vi "Library - Description.vi"(7 "Msg Chain":string, 8 "error in (no error)":errorcluster {"code" format="Error %.0f"}, 10 "Libraries":refnum<class "Library Documentation.lvclass">[](array[class]), 11 "VIDoc Printer - Confluence In":refnum<class "VIDoc Printer - Confluence.lvclass">) -> (0 "error out":errorcluster {"code" format="Error %.0f"}, 3 "VIDoc Printer - Confluence Out":refnum<class "VIDoc Printer - Confluence.lvclass">)   [LabVIEW 2023, in "VIDoc Printer - Confluence.lvlib" / "VIDoc Printer - Confluence.lvclass"]
uses:
  VIDoc Printer - Confluence.lvclass
  C:/projects/DMC/Tooling/Git-Action-Service/Source/Documentation Generation/Printers/Printer/VIDoc Printer.lvclass
  Parsing/Library Documentation/Library Documentation.lvclass
  Parsing/Library Documentation/Library Documentation.lvclass/Library Documentation.ctl
  Parsing/Library Documentation/Get Library Info.vi
  Parsing/Library Documentation/Get Name.vi
  VIDoc Printer - Confluence.lvclass/VIDoc Printer - Confluence.ctl
  Printer/VIDoc Printer.lvclass
  UI Interaction/UI Interaction.lvclass
  C:/projects/DMC/Tooling/Git-Action-Service/Source/Documentation Generation/Printers/Confluence Printer/VIDoc Printer - Confluence.lvclass
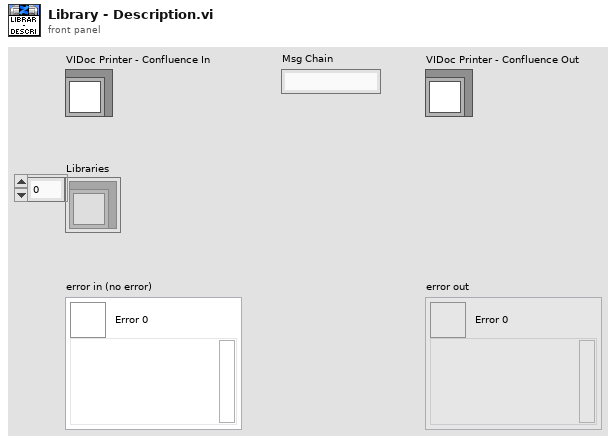
[diagram p1: front panel]
types:
  T1 = typedef "VIDoc Parsing.lvlib/Base Library Info Cluster.ctl" = cluster{"Name":string, "Icon":T2, "Version":cluster{"Major":u16, "Minor":u16, "Fix":u16, "Build":u16}, "Description":string, "Path":path, "Friends":string[], "Library Scope":enum32{"invalid scope", "public", "private", "protected", "community"}, "Qualified Name":string}
  T2 = typedef "imagedata.ctl" = cluster{"image type":i32, "image depth":i32, "image":u8[], "mask":u8[], "colors":u32[], "Rectangle":cluster{"left":i16, "top":i16, "right":i16, "bottom":i16}}
  T3 = enum32{"invalid scope", "public", "private", "protected", "community"}
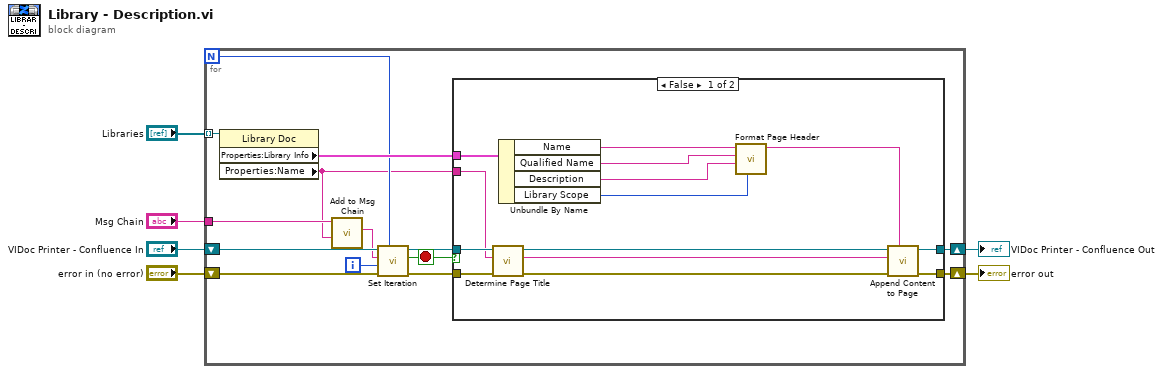
[diagram p0: block diagram]
diagram:
  n1 = for {
    N -> [w12]
    shift-right: [w18] -> w6
    shift-left: "error in (no error)" -> [w15]
    shift-right: [w19] -> w5
    shift-left: "VIDoc Printer - Confluence In" -> [w16]
    tunnel: "Libraries" -> [w20] mode=indexing
    tunnel: "Msg Chain" -> [w10]
    i -> [w11]
    stop <- w7 stop-if-true
    n2 = property class="Library Doc"(reference=w20) -> ("Properties:Library Info"=w17:T1, "Properties:Name"=w9:string)  [unwired: 1 in, 2 out]
    n3 = call "Add to Msg Chain.vi"("New"=w9, "Msg Chain in"=w10) -> ("Msg Chain out"=w8:string)  [unwired: 9 in]
    n4 = call "Set Iteration.vi"("Progress Max"=w12, "error in (no error)"=w15, "Progress Value"=w11, "Message (No Message Update)"=w8, "VIDoc Printer In"=w16) -> ("error out"=w13:errorcluster, "Abort?"=w7:bool, "VIDoc Printer Out"=w14:refnum<class "VIDoc Printer - Confluence.lvclass">)  [unwired: 4 in]
    n5 = case shown="False" w7 {
      tunnel: [w31 w35] -> w19
      tunnel: [w30 w36] -> w18
      tunnel: w17 -> [w29 _]
      tunnel: w14 -> [w27 w35]
      tunnel: w13 -> [w26 w36]
      tunnel: w9 -> [w25 _]
      frame False {
        n6 = call "Determine Page Title.vi"("error in (no error)"=w26, "Name"=w25, "VIDoc Printer - Confluence In"=w27) -> ("error out"=w33:errorcluster, "Page Title"=w34:string, "VIDoc Printer - Confluence Out"=w32:refnum<class "VIDoc Printer - Confluence.lvclass">)  [unwired: 5 in, 1 out]
        n7 = Unbundle By Name(w29) -> ("Name"=w23:string, "Qualified Name"=w22:string, "Description"=w28:string, "Library Scope"=w21:T3)
        n8 = call "Format Page Header.vi"("Library Scope"=w21, "Description"=w28, "Qualified Name"=w22, "Name"=w23) -> ("Text Output"=w24:string)  [unwired: 7 in]
        n9 = call "Append Content to Page.vi"("Page Content"=w24, "error in (no error)"=w33, "Page Title"=w34, "VIDoc Printer - Confluence In"=w32) -> ("error out"=w30:errorcluster, "VIDoc Printer - Confluence Out"=w31:refnum<class "VIDoc Printer - Confluence.lvclass">)  [unwired: 6 in]
      }
      frame True {
      }
    }
  }
  "error out" <- w6
  "VIDoc Printer - Confluence Out" <- w5
